vi "Variant to Variant Attributes.vi"(8 "error in":errorcluster, 9 "Parent is object":bool, 10 "Variant":variant, 11 "Variant with Attributes":variant) -> (0 "error out":errorcluster, 3 "Variant with Attributes":variant)   [LabVIEW 2015, in "JKI JSON Serialization.lvlib" / "JSON Deserializer.lvclass"]
doc: "Re-encodes a <b>Variant</b> of flattened LabVIEW data into attributes of a new <b>Variant with Data as Attributes</b>. \n\nIn this format, scalars and arrays are represented as their respective Variant types while clusters are represented by data of void type, with a variant attribute defined for each member of the object (cluster). LabView uses a hash table to store variant attributes, so the lookup performance is good. Use Get Variant Attribute and cast the appropriate data type to extract data. Note that nested clusters will also have data of void type; their attributes will not be visible until the object is extracted.\n\nThis VI is designed for use in deserializing JSON data where the top-level JSON structure must be an array or an object and duplicate names at the same level are not allowed. Data loss may occur if flattened LabVIEW stuctures containing duplicate names are passed as input."
uses:
  JSON Deserializer.lvclass
  <vilib>/Utility/Data Type/Type Definitions/Data Type.ctl
  <vilib>/Utility/Data Type/NI_Data Type.lvlib
panel:
  out "call chain":string[](array[string])
  out "Type":T1
  out "Name":string
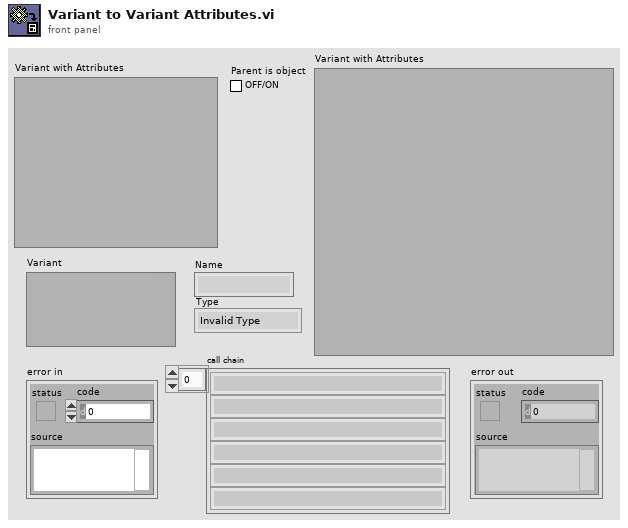
[diagram p1: front panel]
types:
  T1 = typedef "NI_Data Type.lvlib/Data Type.ctl" = enum8{"Invalid Type", "Void", "I8", "I16", "I32", "I64", "U8", "U16", "U32", "U64", "Single Float", "Double Float", "Extended Float", "Single Complex", "Double Complex", "Extended Complex", "Enum U8", "Enum U16", "Enum U32", "Enum U64", "Single Float With Unit", "Double Float With Unit", "Extended Float With Unit", "Single Complex with Unit", "Double Complex with Unit", "Extended Complex with Unit", "Boolean", "String", "Path", "Picture", "Tag", "Array", "Cluster", "Variant", "LV Variant", "Waveform", "Timestamp", "Digital Waveform", "Digital Data", "ExpressData", "Refnum", "External Data", "VI", "Poly VI", "LabVIEW Class Instance", "Fixed Point"}
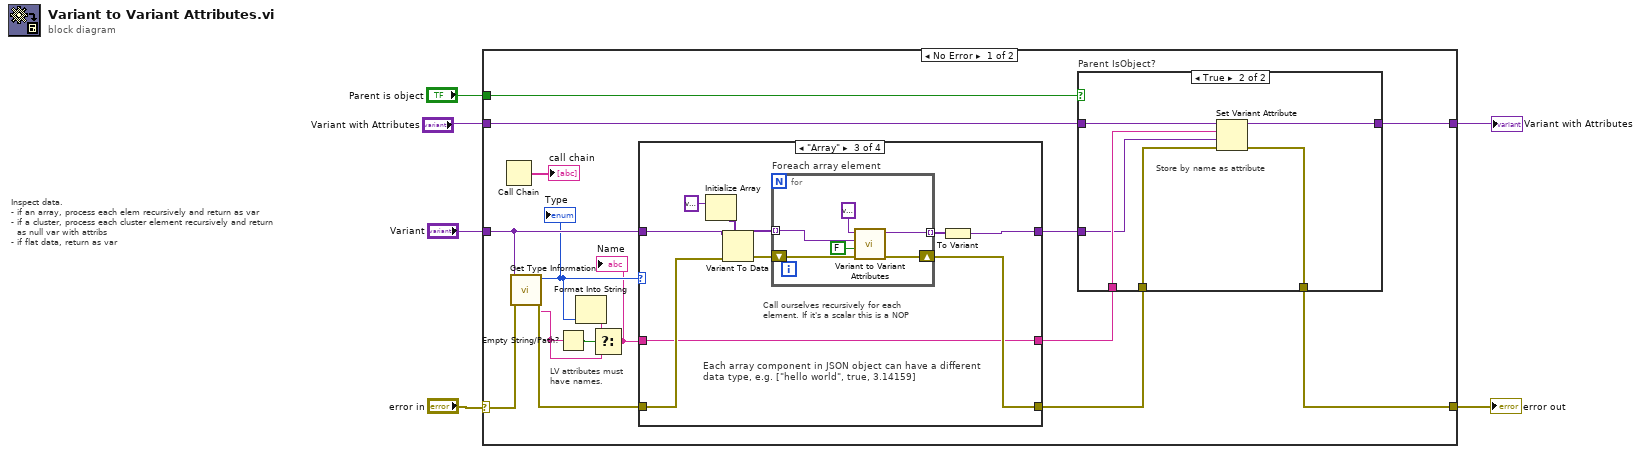
[diagram p0: block diagram]
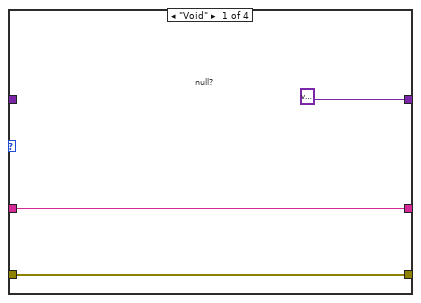
[diagram p3: hidden frame]
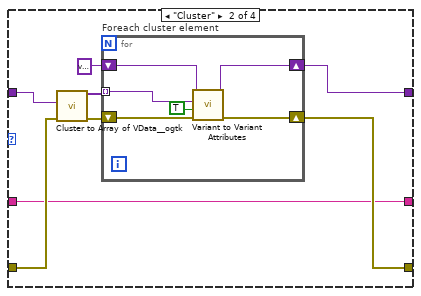
[diagram p4: hidden frame]
diagram:
  # "Inspect data.\n- if an array, process each elem recursively and return as var\n- if a cluster, process each cluster element recursively and return\n  as null var with attribs\n- if flat data, return as var"
  n1 = case shown="No Error" "error in" {
    selector: "error in" -> [w22 w67]
    tunnel: [w8 w67] -> w5
    tunnel: "Variant" -> [w20 _]
    tunnel: [w13 _] -> w3
    tunnel: "Variant with Attributes" -> [w7 _]
    tunnel: "Parent is object" -> [w12 _]
    frame No Error {
      # "LV attributes must\nhave names."
      n2 = Call Chain() -> (call chain=→"call chain":string[])
      n3 = call <vilib>:"Get Type Information.vi"("error in (no error)"=w22, "Variant"=w20) -> ("error out"=w21:errorcluster, "Name"=w16:string, "Type"=w18:T1)  [unwired: 5 in, 2 out]
      "Type" <- w18
      n4 = Empty String/Path?(string/path=w16) -> (empty?=w19:bool)
      n5 = Format Into String(w18) -> (resulting string=w17:string)  [unwired: 3 in, 1 out]
      n6 = Select(t=w17, s=w19, f=w16) -> (s? t:f=w15:string)
      "Name" <- w15
      n7 = case shown="\"Array\"" w18 {
        tunnel: [w33 w35 w52 w66] -> w9
        tunnel: w21 -> [w33 w41 w57 w66]
        tunnel: w20 -> [_ w39 w50 w65]
        tunnel: w15 -> [w32 w34 w48 w64]
        tunnel: [variant w36 w49 w65] -> w11
        tunnel: [w32 w34 w48 w64] -> w10
        frame "Void" {
          # "null?"
        }
        frame "Cluster" {
          n8 = call <userlib>:"Cluster to Array of VData__ogtk.vi"("error in (no error)"=w41, "Cluster"=w39) -> ("error out"=w40:errorcluster, "Array of VData"=w38:variant[])  [unwired: 8 in]
          n9 = for "Foreach cluster element" {
            tunnel: w38 -> [w45] mode=indexing
            shift-right: [w46] -> w36
            shift-left: variant -> [w47]
            shift-right: [w43] -> w35
            shift-left: w40 -> [w44]
            n10 = call "Variant to Variant Attributes.vi"("error in"=w44, "Parent is object"=TRUE, "Variant"=w45, "Variant with Attributes"=w47) -> ("error out"=w43:errorcluster, "Variant with Attributes"=w46:variant)  [unwired: 6 in]
          }
        }
        frame "Array" {
          # "Call ourselves recursively for each\nelement. If it's a scalar this is a NOP"
          # "Each array component in JSON object can have a different\ndata type, e.g. [\"hello world\", true, 3.14159]"
          n11 = Initialize Array(variant) -> (w54:variant[])  [unwired: 1 in]
          n12 = Variant To Data(error in=w57, type=w54, Variant=w50) -> (data=w53:variant[], error out=w56:errorcluster)
          n13 = for "Foreach array element" {
            tunnel: w53 -> [w61] mode=indexing
            shift-right: [w63] -> w52
            shift-left: w56 -> [w59]
            tunnel: [w62] -> w51 mode=indexing
            n14 = call "Variant to Variant Attributes.vi"("error in"=w59, "Parent is object"=FALSE, "Variant"=w61, "Variant with Attributes"=variant) -> ("error out"=w63:errorcluster, "Variant with Attributes"=w62:variant)  [unwired: 6 in]
          }
          n15 = To Variant(anything=w51) -> (Variant=w49:variant)
        }
        frame Default {
          # "scalar value"
        }
      }
      n16 = case "Parent IsObject?" shown="True" w12 {
        tunnel: w7 -> [_ w30]
        tunnel: [w24 w29] -> w13
        tunnel: w10 -> [_ w28]
        tunnel: w11 -> [w24 w27]
        tunnel: w9 -> [w23 w26]
        tunnel: [w23 w25] -> w8
        frame False {
          # "scalar or member of array"
        }
        frame True {
          # "Store by name as attribute"
          n17 = Set Variant Attribute(Variant=w30, name=w28, value=w27, error in=w26) -> (Variant out=w29:variant, error out=w25:errorcluster)  [unwired: 1 out]
        }
      }
    }
    frame Error {
    }
  }
  "error out" <- w5
  "Variant with Attributes" <- w3
